vi "MeasureEventCallback.vi"(4 "?":refnum<vi>, 5 "Event Data":cluster{"sender":refnum<k24>, "e":refnum<k24>}, 6 "Control Ref":refnum<k24>, 7 "Event Common Data":T1) -> ()   [LabVIEW 2014]
uses:
  C:/Users/ThomasNelson/Projects/examples/libraries/bin/visual .net/KClmtrWrapper.dll
  libraries/bin/visual .net/KClmtrWrapper.dll
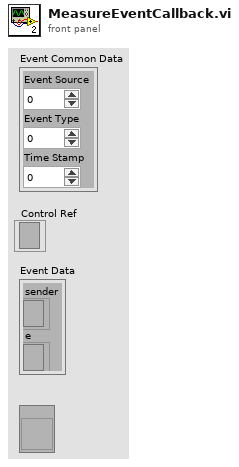
[diagram p1: front panel]
types:
  T1 = cluster{"Event Source":i32, "Event Type":u32, "Time Stamp":u32}
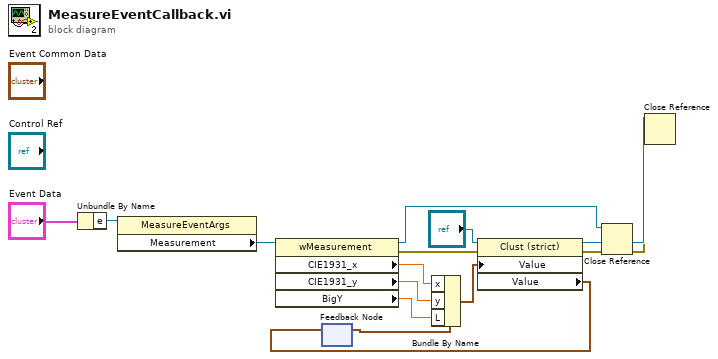
[diagram p0: block diagram]
diagram:
  n1 = Unbundle By Name("Event Data") -> ("e"=w14:refnum<k24>)
  n2 = property class="MeasureEventArgs"(reference=w14) -> ("Measurement"=w9:refnum<k24>)  [unwired: 1 in, 2 out]
  n3 = property class="wMeasurement"(reference=w9) -> (reference out=w5:refnum<k24>, error out=w3:errorcluster, "CIE1931_x"=w8:dbl, "CIE1931_y"=w7:dbl, "BigY"=w6:dbl)  [unwired: 1 in]
  n4 = feedback #1() -> (w10:cluster{"x":dbl, "L":dbl, "y":dbl})  [unwired: 1 in]
  n5 = Bundle By Name(cluster=w10, "x"=w8, "y"=w7, "L"=w6) -> (w12:cluster{"x":dbl, "L":dbl, "y":dbl})
  n6 = property class="Clust (strict)"(reference="?", error in=w3, "Value"=w12) -> (reference out=w2:refnum<vi>, error out=w4:errorcluster, "Value"=w11:cluster{"x":dbl, "L":dbl, "y":dbl})
  n7 = feedback-in #1(w11) -> ()
  n8 = Close Reference(reference=w5, error in (no error)=w4) -> (error out=w1:errorcluster)
  n9 = Close Reference(reference=w2, error in (no error)=w1) -> ()  [unwired: 1 out]
